vi "Read Error indices mapping.vi"(8 "error in (no error)":errorcluster, 11 "Error Manager in":refnum<class "Error Manager.lvclass">) -> (0 "error out":errorcluster, 2 "Error indices mapping":map{i32, i32}(c390), 3 "Error Manager out":refnum<class "Error Manager.lvclass">)   [LabVIEW 2026, in "TALOS.lvlib" / "Error Manager.lvlib" / "Error Manager.lvclass"]
uses:
  Error Manager.lvclass
  Error Manager.lvclass/Error Manager.ctl
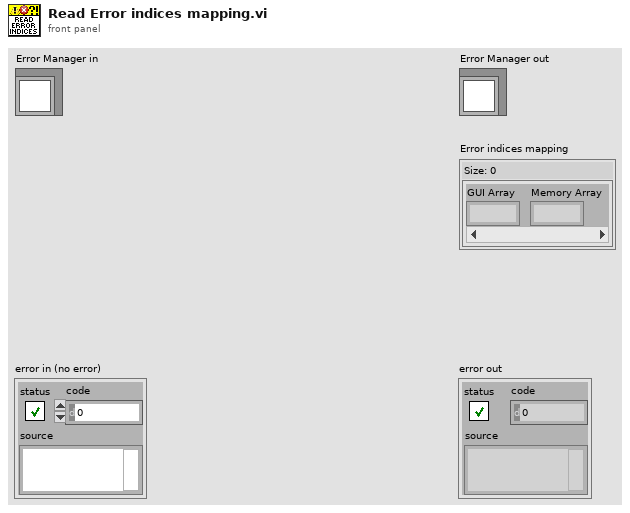
[diagram p1: front panel]
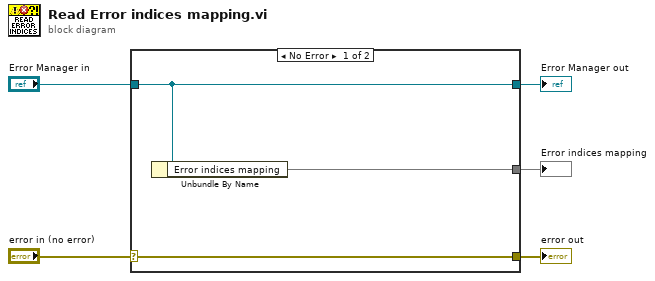
[diagram p0: block diagram]
diagram:
  n1 = case shown="No Error" "error in (no error)" {
    selector: "error in (no error)" -> [w8 w9]
    tunnel: [w8 w9] -> w4
    tunnel: [w7 w10] -> w2
    tunnel: "Error Manager in" -> [w7 w10]
    tunnel: [w6 _] -> w1
    frame No Error {
      n2 = Unbundle By Name(w7) -> ("Error indices mapping"=w6:map{i32, i32})
    }
    frame Error {
    }
  }
  "error out" <- w4
  "Error Manager out" <- w2
  "Error indices mapping" <- w1
